vi "S2DS_Change direction.vi"(3 "X sweep direction":refnum<vi>, 4 "Y sweep direction":refnum<vi>, 5 "Change y direction?":bool, 6 "Change x direction?":bool, 8 "Scan parameters  in":T1 {"Y data taking" items=["in both direction", "in up direction only", "in down direction only"]; "X data taking" items=["in both direction", "in up direction only", "in down direction only"]}) -> (0 "Scan over?":bool, 1 "Scan parameters out":T1 {"Y data taking" items=["in both direction", "in up direction only", "in down direction only"]; "X data taking" items=["in both direction", "in up direction only", "in down direction only"]}, 2 "Change color":bool)   [LabVIEW 2025]
uses:
  TYPE DEFS/S2DS_Sweep Info.ctl
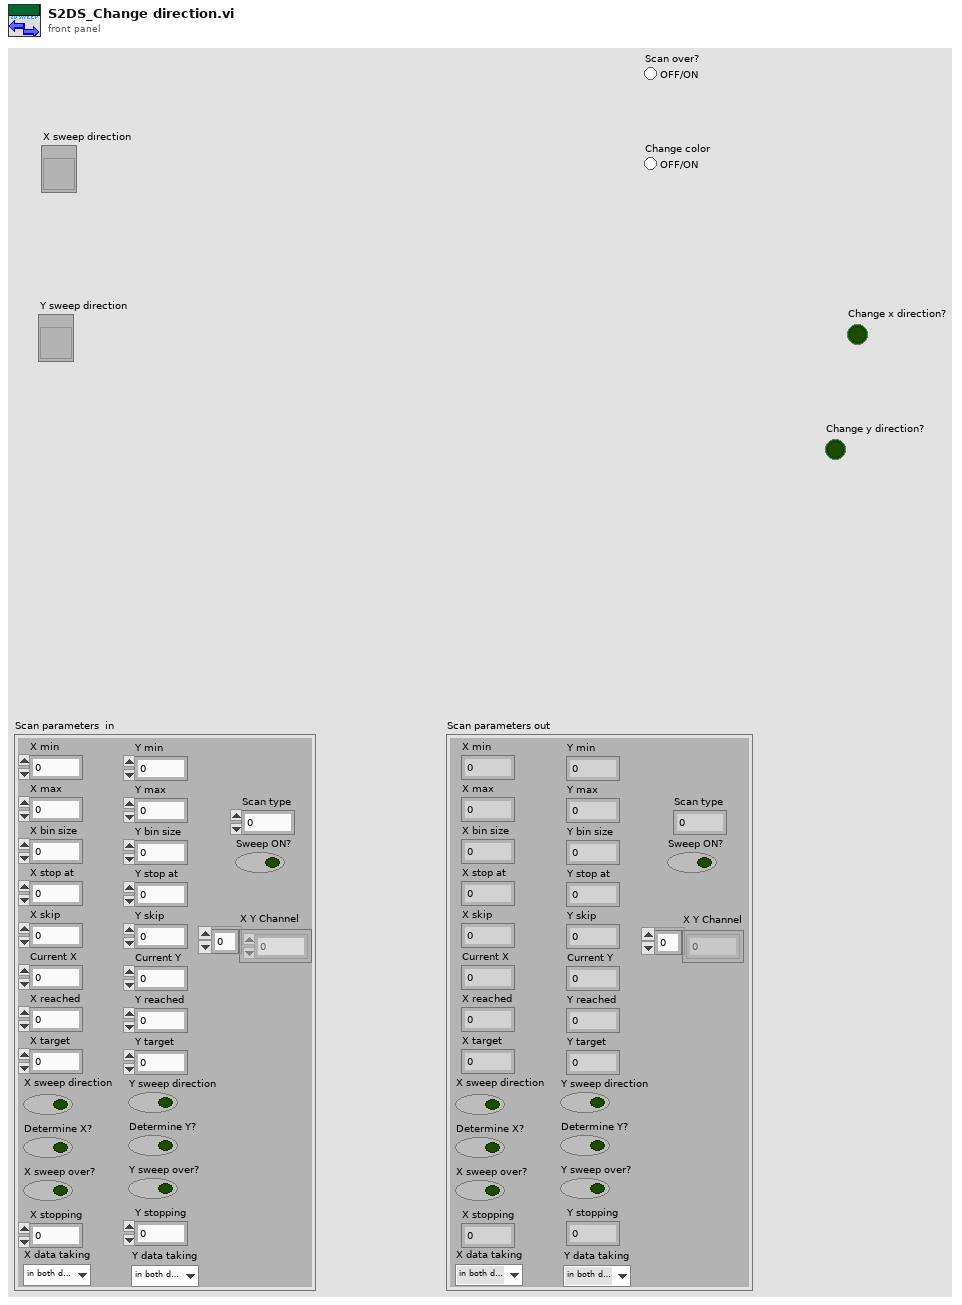
[diagram p1: front panel]
types:
  T1 = typedef "S2DS_Sweep Info.ctl" = cluster{"X min":ext, "X max":dbl, "Y min":dbl, "Y max":dbl, "X bin size":dbl, "Y bin size":dbl, "X stop at":dbl, "Y stop at":dbl, "X skip":u64, "Y skip":u64, "Current X":dbl, "Current Y":dbl, "X reached":i32, "Y reached":i32, "X target":dbl, "Y target":dbl, "Sweep ON?":bool, "X sweep direction":bool, "Y sweep direction":bool, "Determine X?":bool, "Determine Y?":bool, "X sweep over?":bool, "Y sweep over?":bool, "Scan type":i32, "X stopping":i32, "Y stopping":i32, "X Y Channel":u16[], "X data taking":u16, "Y data taking":u16}
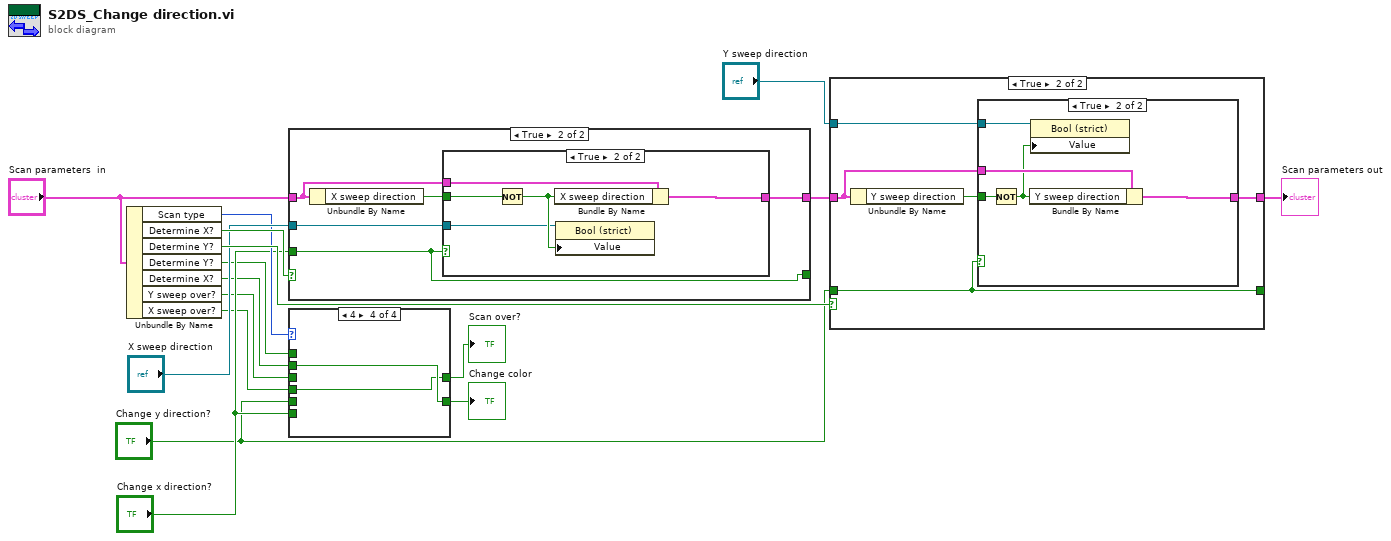
[diagram p0: block diagram]
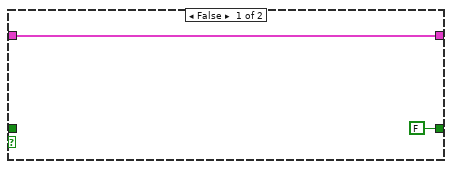
[diagram p5: hidden frame]
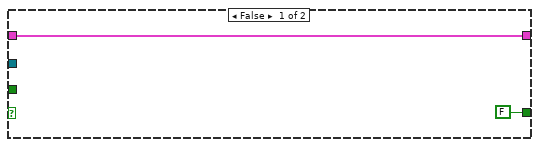
[diagram p7: hidden frame]
diagram:
  n1 = Unbundle By Name("Scan parameters  in") -> ("Scan type"=w9:i32, "Determine X?"=w14:bool, "Determine Y?"=w13:bool, "Determine Y?"=w5:bool, "Determine X?"=w4:bool, "Y sweep over?"=w1:bool, "X sweep over?"=w2:bool)
  n2 = case shown="True" w14 {
    tunnel: "Scan parameters  in" -> [w17 w22]
    tunnel: [FALSE w19] -> _
    tunnel: [w17 w21] -> w15
    tunnel: "X sweep direction" -> [_ w20]
    tunnel: "Change x direction?" -> [_ w19]
    frame False {
    }
    frame True {
      n3 = Unbundle By Name(w22) -> ("X sweep direction"=w23:bool)
      n4 = case shown="True" w19 {
        tunnel: w23 -> [_ w29]
        tunnel: w22 -> [w24 w28]
        tunnel: [w24 w26] -> w21
        tunnel: w20 -> [_ w25]
        frame False {
        }
        frame True {
          n5 = Not(x=w29) -> (.not. x?=w27:bool)
          n6 = Bundle By Name(cluster=w28, "X sweep direction"=w27) -> (w26:T1)
          n7 = property on="Property Node" class="Bool (strict)"(reference=w25, "Value"=w27) -> ()  [unwired: 1 in, 2 out]
        }
      }
    }
  }
  n8 = case shown="4" w9 {
    tunnel: [w31 w33 w35 w37] -> w7
    tunnel: "Change x direction?" -> [w31 _ _ _]
    tunnel: "Change y direction?" -> [_ w33 _ _]
    tunnel: w5 -> [_ _ w35 _]
    tunnel: w4 -> [_ _ _ w37]
    tunnel: [w30 w32 w34 w36] -> w3
    tunnel: w2 -> [w30 _ _ w36]
    tunnel: w1 -> [_ w32 w34 _]
    frame 1, Default {
    }
    frame 2 {
    }
    frame 3 {
    }
    frame 4 {
    }
  }
  "Change color" <- w7
  "Scan over?" <- w3
  n9 = case shown="True" w13 {
    tunnel: w15 -> [w38 w43]
    tunnel: [FALSE w40] -> _
    tunnel: [w38 w42] -> w10
    tunnel: "Y sweep direction" -> [_ w41]
    tunnel: "Change y direction?" -> [_ w40]
    frame False {
    }
    frame True {
      n10 = Unbundle By Name(w43) -> ("Y sweep direction"=w44:bool)
      n11 = case shown="True" w40 {
        tunnel: w44 -> [_ w50]
        tunnel: w43 -> [w45 w49]
        tunnel: [w45 w47] -> w42
        tunnel: w41 -> [_ w46]
        frame False {
        }
        frame True {
          n12 = Not(x=w50) -> (.not. x?=w48:bool)
          n13 = Bundle By Name(cluster=w49, "Y sweep direction"=w48) -> (w47:T1)
          n14 = property on="Property Node" class="Bool (strict)"(reference=w46, "Value"=w48) -> ()  [unwired: 1 in, 2 out]
        }
      }
    }
  }
  "Scan parameters out" <- w10
